vi "GetNeighbors.vi"(8 "error in (no error)":errorcluster, 9 "get predecessors (F)":bool, 10 "AbstractMapNode Ref":refnum<data-value>, 11 "WorldMap in":refnum<class "NI_Robotics_OccupancyGridWorldMap.lvclass">) -> (0 "error out":errorcluster, 1 "EdgeCost":dbl[](array[numeric]), 2 "Successors":refnum<data-value>[](array[refnum]), 3 "WorldMap out":refnum<class "NI_Robotics_OccupancyGridWorldMap.lvclass">)   [LabVIEW 2017, in "NI_Robotics_OccupancyGridWorldMap.lvclass"]
uses:
  <vilib>/robotics/Navigation/shared/WorldMap/OccupancyGridWorldMap/NI_Robotics_OccupancyGridWorldMap.lvclass
  <vilib>/robotics/Navigation/shared/MapNode/AbstractMapNode/NI_Robotics_AbstractMapNode.lvclass
  <vilib>/robotics/Navigation/shared/MapNode/OccupancyGridNode/NI_Robotics_OccupancyGridMapNode.lvclass
  c:/Program Files (x86)/National Instruments/LabVIEW 2017/vi.lib/robotics/Navigation/shared/MapNode/AbstractMapNode/NI_Robotics_AbstractMapNode.lvclass
  <vilib>/robotics/Navigation/shared/WorldMap/OccupancyGridWorldMap/NI_Robotics_OccupancyGridWorldMap.lvclass/NI_Robotics_OccupancyGridWorldMap.ctl
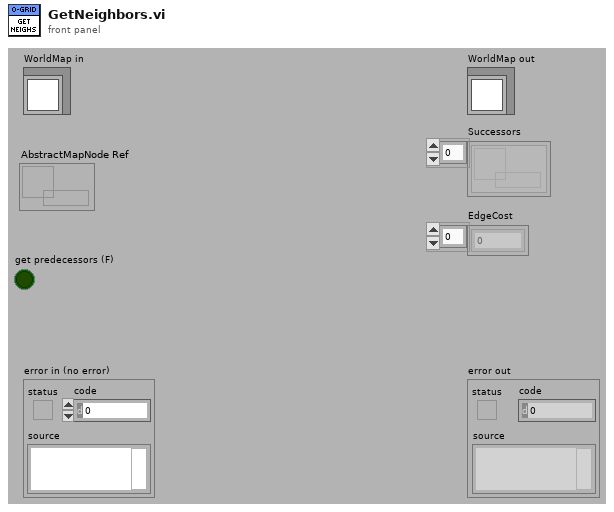
[diagram p1: front panel]
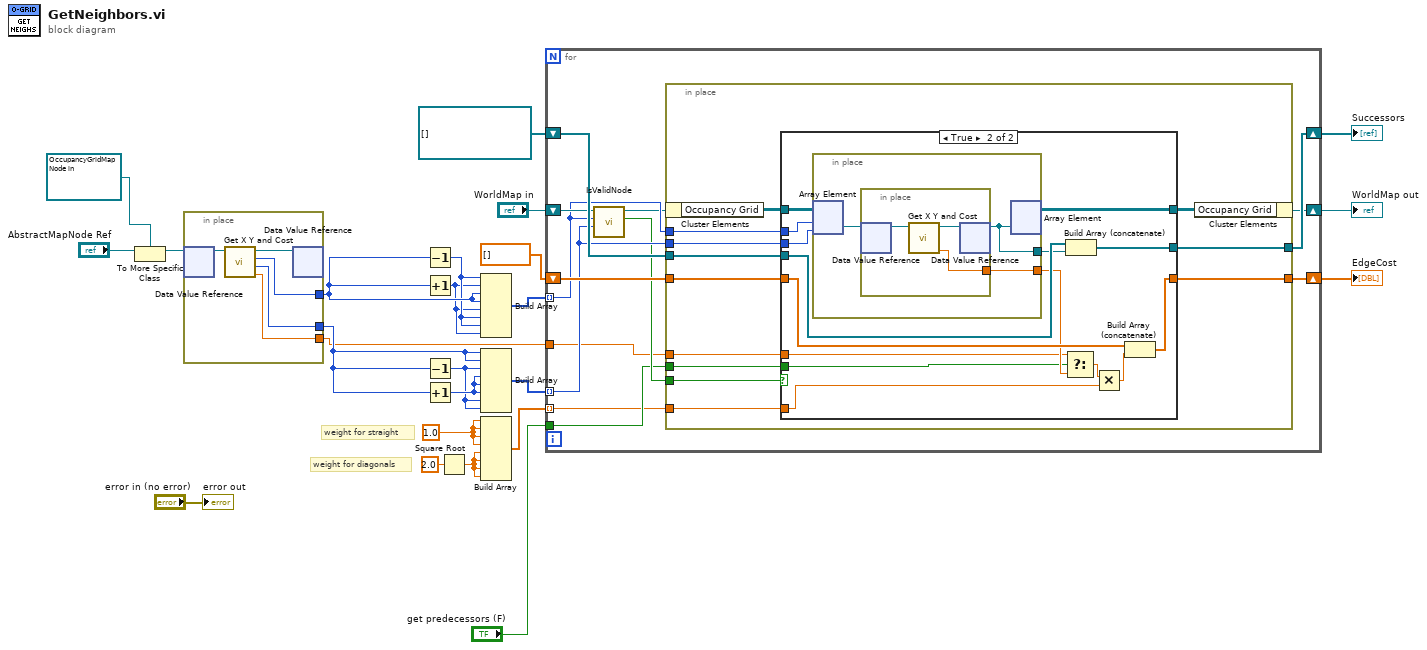
[diagram p0: block diagram]
diagram:
  w2 = 1.0
  # "weight for diagonals"
  # "weight for straight"
  n1 = To More Specific Class(target class=refnum<data-value> refnum ("data value reference"), reference="AbstractMapNode Ref") -> (specific class reference=w24:refnum<data-value>)  [unwired: 1 in, 1 out]
  n2 = in-place {
    in-place-border: [w27] -> w13
    in-place-border: [w26] -> w14
    in-place-border: [w25] -> w9
    n3 = in-place-dvr #1(w24) -> (w29:refnum<class "NI_Robotics_OccupancyGridMapNode.lvclass">)  [unwired: 1 out]
    n4 = call-dynamic "Get X Y and Cost.vi"("OccupancyGridMapNode in"=w29) -> ("Cost"=w25:dbl, "y"=w26:i32, "x"=w27:i32, "OccupancyGridMapNode out"=w28:refnum<class "NI_Robotics_OccupancyGridMapNode.lvclass">)  [unwired: 7 in]
    n5 = in-place-dvr #1(w28) -> ()  [unwired: 2 out]
  }
  n6 = Decrement(x=w13) -> (x-1=w6:i32)
  n7 = Increment(x=w13) -> (x+1=w5:i32)
  n8 = Decrement(x=w14) -> (x-1=w7:i32)
  n9 = Increment(x=w14) -> (x+1=w8:i32)
  n10 = Square Root(x=2.0) -> (sqrt(x)=w1:dbl)
  n11 = Build Array(w6, w5, w13, w13, w5, w6, w6, w5) -> (w21:i32[])
  n12 = Build Array(w14, w14, w7, w8, w8, w8, w7, w7) -> (w20:i32[])
  n13 = Build Array(w2, w2, w2, w2, w1, w1, w1, w1) -> (w3:dbl[])
  n14 = for {
    tunnel: w21 -> [w37] mode=indexing
    tunnel: w20 -> [w36] mode=indexing
    shift-right: [w41] -> w19
    shift-left: refnum<data-value>[] [] -> [w42]
    shift-right: [w39] -> w18
    shift-left: dbl[] [] -> [w40]
    shift-right: [w33] -> w11
    shift-left: "WorldMap in" -> [w38]
    tunnel: "get predecessors (F)" -> [w32]
    tunnel: w9 -> [w31]
    tunnel: w3 -> [w30] mode=indexing
    n15 = call <vilib>:"IsValidNode.vi"("y"=w36, "x"=w37, "OccupancyGridWorldMap in"=w38) -> ("Valid"=w35:bool, "OccupancyGridWorldMap out"=w34:refnum<class "NI_Robotics_OccupancyGridWorldMap.lvclass">)  [unwired: 7 in]
    n16 = in-place {
      in-place-border: w42 -> [w54]
      in-place-border: [w53] -> w41
      in-place-border: w40 -> [w52]
      in-place-border: [w51] -> w39
      in-place-border: w37 -> [w50]
      in-place-border: w36 -> [w49]
      in-place-border: w35 -> [w48]
      in-place-border: w32 -> [w45]
      in-place-border: w31 -> [w44]
      in-place-border: w30 -> [w43]
      n17 = in-place-cluster #2(w34) -> ("Occupancy Grid"=w47:refnum<data-value>[][])
      n18 = case shown="True" w48 {
        tunnel: w47 -> [w55 w72]
        tunnel: w50 -> [_ w71]
        tunnel: w49 -> [_ w70]
        tunnel: [w55 w69] -> w46
        tunnel: w54 -> [w57 w68]
        tunnel: [w57 w66] -> w53
        tunnel: w52 -> [w56 w65]
        tunnel: [w56 w64] -> w51
        tunnel: w45 -> [_ w62]
        tunnel: w44 -> [_ w61]
        tunnel: w43 -> [_ w58]
        frame False {
        }
        frame True {
          n19 = in-place {
            in-place-border: [w74] -> w63
            in-place-border: [w73] -> w67
            n20 = in-place-array #3(w72, w71, w70) -> (w75:refnum<data-value>)
            n21 = in-place {
              in-place-border: [w76] -> w74
              n22 = in-place-dvr #4(w75) -> (w78:refnum<class "NI_Robotics_OccupancyGridMapNode.lvclass">)  [unwired: 1 out]
              n23 = call-dynamic "Get X Y and Cost.vi"("OccupancyGridMapNode in"=w78) -> ("Cost"=w76:dbl, "OccupancyGridMapNode out"=w77:refnum<class "NI_Robotics_OccupancyGridMapNode.lvclass">)  [unwired: 7 in, 2 out]
              n24 = in-place-dvr #4(w77) -> (w73:refnum<data-value>)  [unwired: 1 out]
            }
            n25 = in-place-array #3(w73) -> (w69:refnum<data-value>[][])  [unwired: 2 out]
          }
          n26 = Select(t=w61, s=w62, f=w63) -> (s? t:f=w60:dbl)
          n27 = Build Array (concatenate)(w68, w67) -> (w66:refnum<data-value>[])
          n28 = Multiply(x=w60, y=w58) -> (x*y=w59:dbl)
          n29 = Build Array (concatenate)(w65, w59) -> (w64:dbl[])
        }
      }
      n30 = in-place-cluster #2("Occupancy Grid"=w46) -> (w33:refnum<class "NI_Robotics_OccupancyGridWorldMap.lvclass">)
    }
  }
  "WorldMap out" <- w11
  "Successors" <- w19
  "EdgeCost" <- w18
  "error out" <- "error in (no error)"
